vi "RM-go-home.vi"(8 "error in (no error)":errorcluster, 11 "MB_Master_Serial输入":refnum<class "MB_Master_Serial.lvclass">) -> (0 "error out":errorcluster, 3 "MB_Master_Serial输出":refnum<class "MB_Master_Serial.lvclass">)   [LabVIEW 2014]
uses:
  <vilib>/Plasmionique/MB Master/MB_Master_Serial/MB_Master_Serial.lvclass
  <vilib>/Plasmionique/MB Master/MB Master.lvlib
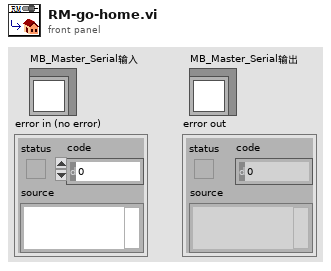
[diagram p1: front panel]
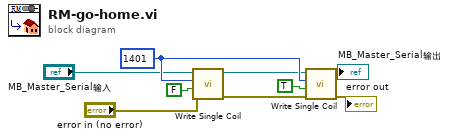
[diagram p0: block diagram]
diagram:
  w9 = u16 1401 ("address")
  n1 = call <vilib>:"Write Single Coil.vi"("error in (no error)"="error in (no error)", "value"=FALSE, "address"=w9, "MB session in"="MB_Master_Serial输入") -> ("error out"=w5:errorcluster, "MB session out"=w6:refnum<class "MB_Master_Serial.lvclass">)  [unwired: 6 in]
  n2 = call <vilib>:"Write Single Coil.vi"("error in (no error)"=w5, "value"=TRUE, "address"=w9, "MB session in"=w6) -> ("error out"=→"error out":errorcluster, "MB session out"=→"MB_Master_Serial输出":refnum<class "MB_Master_Serial.lvclass">)  [unwired: 6 in]
